vi "Construct.vi"(8 "error in (no error)":errorcluster, 11 "SolutionBuilder in":refnum<class "SolutionBuilder.lvclass">) -> (0 "error out":errorcluster, 3 "SolutionBuilder out":refnum<class "SolutionBuilder.lvclass">)   [LabVIEW 2020, in "SolutionBuilder.lvlib" / "SolutionBuilder.lvclass"]
uses:
  SolutionBuilder.lvclass
  SolutionBuilder.lvclass/SolutionBuilder.ctl
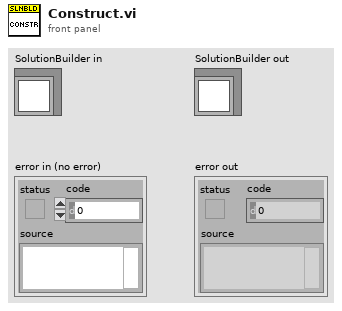
[diagram p1: front panel]
types:
  T1 = typedef "SolutionBuilder.lvlib/SolutionBuilder.lvclass/Options.ctl" = cluster{"Path":path, "Preview?":bool, "Quiet?":bool, "Show help?":bool}
  T2 = typedef "SolutionBuilder.lvlib/SolutionBuilder.lvclass/ItemInfo.ctl" = map{string, T3}
  T3 = typedef "SolutionBuilder.lvlib/SolutionBuilder.lvclass/ProjectInfo.ctl" = cluster{"Deps":set{string}, "FileInfo":T4}
  T4 = typedef "SolutionBuilder.lvlib/SolutionBuilder.lvclass/FileInfo.ctl" = cluster{"Library ref":refnum<vi>, "Target path":path, "Source name":string, "Build spec name":string}
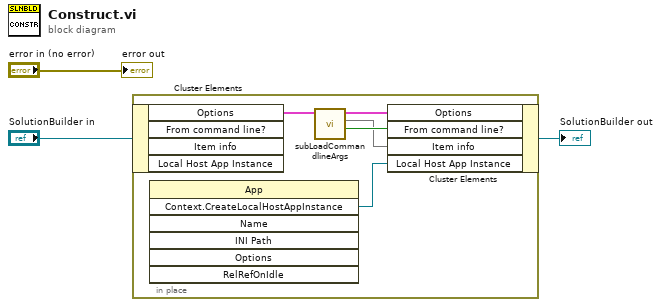
[diagram p0: block diagram]
diagram:
  n1 = in-place {
    n2 = in-place-cluster #1("SolutionBuilder in") -> ("Options"=w8:T1)  [unwired: 3 out]
    n3 = invoke class="App" method="Context.CreateLocalHostAppInstance"() -> ("Create Context"=w5:refnum<vi>)  [unwired: 7 in, 6 out]
    n4 = call "subLoadCommandlineArgs.vi"("Options in"=w8) -> ("From command line?"=w6:bool, "Item info"=w4:T2, "Options"=w7:T1)  [unwired: 7 in, 1 out]
    n5 = in-place-cluster #1("Options"=w7, "From command line?"=w6, "Item info"=w4, "Local Host App Instance"=w5) -> (→"SolutionBuilder out":refnum<class "SolutionBuilder.lvclass">)
  }
  "error out" <- "error in (no error)"
